vi "Normalized to Encoder Velocity.vi"(8 "Enum":T1(ring), 11 "ft/s":dbl) -> (3 "Output":dbl)   [LabVIEW 2019]
panel:
  in  "y":dbl=0.85 format="%#_13g"
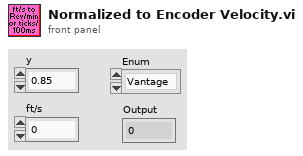
[diagram p1: front panel]
types:
  T1 = enum16{"Vantage", "Mule", "Linda/Sophie", "Rose/Maple"}
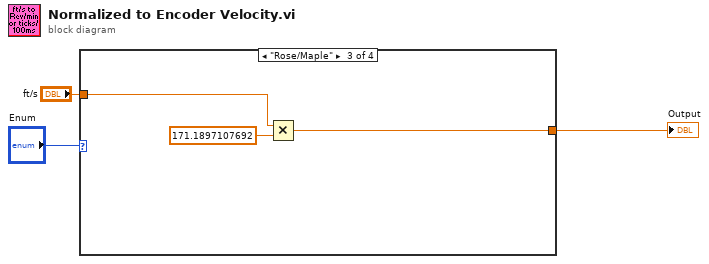
[diagram p0: block diagram]
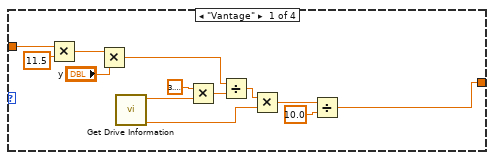
[diagram p2: hidden frame]
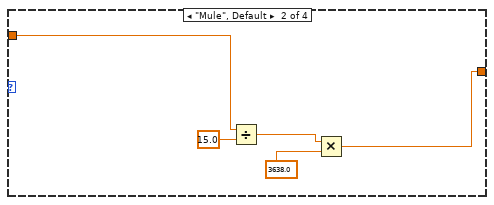
[diagram p3: hidden frame]
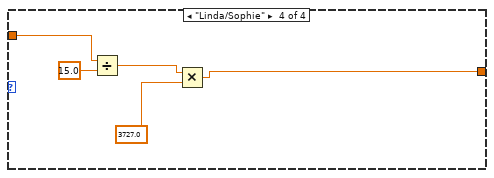
[diagram p4: hidden frame]
diagram:
  n1 = case shown="\"Rose/Maple\"" "Enum" {
    tunnel: "ft/s" -> [w16 w19 w24 w29]
    tunnel: [w4 w18 w23 w25] -> w1
    frame "Vantage" {
      n2 = Multiply(x=w16, y=11.5) -> (x*y=w7:dbl)
      n3 = Multiply(x=w7, y="y") -> (x*y=w5:dbl)
      n4 = call "Get Drive Information.vi"() -> ("Ticks/Revolution"=w8:dbl, "Wheel Diameter"=w9:dbl)  [unwired: 10 in]
      n5 = Multiply(x=3.141592653589793, y=w9) -> (x*y=w13:dbl)
      n6 = Divide(x=w5, y=w13) -> (x/y=w12:dbl)
      n7 = Multiply(x=w12, y=w8) -> (x*y=w11:dbl)
      n8 = Divide(x=w11, y=10.0) -> (x/y=w4:dbl)
    }
    frame "Mule", Default {
      n9 = Divide(x=w19, y=15.0) -> (x/y=w20:dbl)
      n10 = Multiply(x=w20, y=3638.0 ("y 2")) -> (x*y=w18:dbl)
    }
    frame "Rose/Maple" {
      n11 = Multiply(x=w24, y=171.1897107692) -> (x*y=w23:dbl)
    }
    frame "Linda/Sophie" {
      n12 = Divide(x=w29, y=15.0) -> (x/y=w27:dbl)
      n13 = Multiply(x=w27, y=3727.0 ("Scaling")) -> (x*y=w25:dbl)
    }
  }
  "Output" <- w1
